vi "抓圓_new.vi"(0 "Image In":T6, 1 "ROI":T5, 4 "Gap":i32=10 min=1 max=300, 5 "error In":errorcluster, 6 "Process":T8(ring), 7 "Options":T3={"Search Direction"=0, "Edge Options"={"Edge Polarity"=0, "Kernel Size"=3, "Width"=3, "Minimum Edge Strength"=10.0, "Interpolation Type"=enum."Bilinear Fixed", "Data Processing Method"=enum."Average"}, "Show Search Area"=FALSE, "Show Search Lines"=FALSE, "Show Edges Found"=FALSE, "Show Result"=TRUE, "Search Area Color"=65280, "Search Lines Color"=255, "Edge Locations Color"=16776960, "Result Color"=16711680, "Overlay Group Name"=""} {"Edge Options"."Edge Polarity" items=["All Edges", "Rising Edges", "Falling Edges"]; "Edge Options"."Minimum Edge Strength" format="%.2f"; "Edge Options"."Width" step=2; "Edge Options"."Kernel Size" step=2; "Search Direction" items=["Outer to Inner", "Inner to Outer"]}, 8 "Point Diameter (5)":u32=5 min=3 max=1000, 10 "Optimized Mode":bool=TRUE) -> (13 "Ellipse":T7 {"Minor Axis"."Point 2"."Y" format="%.2f"; "Minor Axis"."Point 2"."X" format="%.2f"; "Minor Axis"."Point 1"."Y" format="%.2f"; "Minor Axis"."Point 1"."X" format="%.2f"; "Major Axis"."Point 2"."Y" format="%.2f"; "Major Axis"."Point 2"."X" format="%.2f"; "Major Axis"."Point 1"."Y" format="%.2f"; "Major Axis"."Point 1"."X" format="%.2f"; "Center"."Y" format="%.2f"; "Center"."X" format="%.2f"}, 14 "Imag e Out":T6, 15 "Line Profile":dbl[][](graph), 19 "error out":errorcluster)   [LabVIEW 2015]
uses:
  <vilib>/vision/Image Controls.llb/IMAQ Image.ctl
  <vilib>/vision/Measure.llb/Edge Options.ctl
  <vilib>/vision/Measure.llb/Edge Polarity.ctl
  <vilib>/vision/NI_Vision_Development_Module.lvlib
panel:
  in  "Coordinate System":T4 {"Measurement System"."Axis Reference" items=["Direct", "Indirect"]; "Measurement System"."Angle (deg)" format="%.2f"; "Measurement System"."Origin"."Y" format="%.2f"; "Measurement System"."Origin"."X" format="%.2f"; "Reference System"."Axis Reference" items=["Direct", "Indirect"]; "Reference System"."Angle (deg)" format="%.2f"; "Reference System"."Origin"."Y" format="%.2f"; "Reference System"."Origin"."X" format="%.2f"}
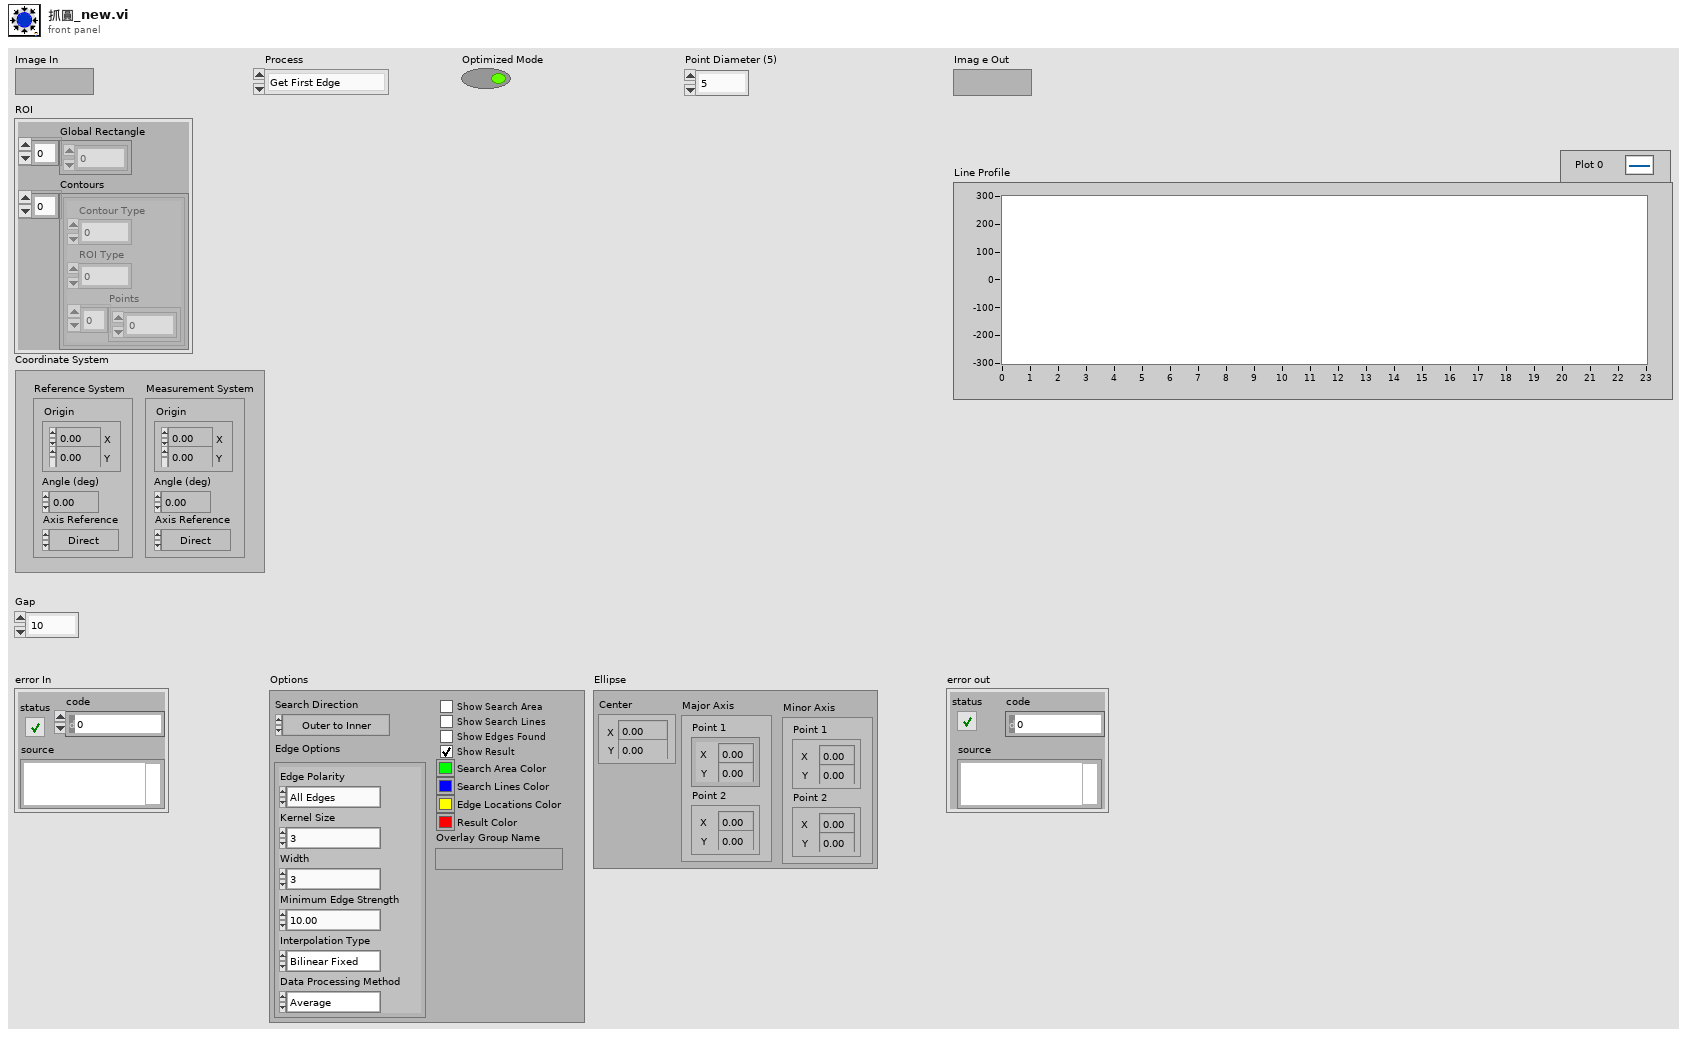
[diagram p1: front panel]
types:
  T1 = typedef "Edge Options.ctl" = cluster{"Edge Polarity":T2, "Kernel Size":u32, "Width":u32, "Minimum Edge Strength":sgl, "Interpolation Type":enum32{"Zero Order", "Bilinear", "Quadratic", "Cubic", "Bilinear Fixed"}, "Data Processing Method":enum32{"Average", "Median"}}
  T2 = typedef "Edge Polarity.ctl" = u32
  T3 = cluster{"Search Direction":u32, "Edge Options":T1, "Show Search Area":bool, "Show Search Lines":bool, "Show Edges Found":bool, "Show Result":bool, "Search Area Color":u32, "Search Lines Color":u32, "Edge Locations Color":u32, "Result Color":u32, "Overlay Group Name":string}
  T4 = typedef "IMAQ Coordinate System" = cluster{"Reference System":cluster{"Origin":cluster{"X":sgl, "Y":sgl}, "Angle (deg)":sgl, "Axis Reference":u32}, "Measurement System":cluster{"Origin":cluster{"X":sgl, "Y":sgl}, "Angle (deg)":sgl, "Axis Reference":u32}}
  T5 = cluster{"Global Rectangle":i32[], "Contours":cluster{"Contour Type":u32, "ROI Type":u32, "Points":i32[]}[]}
  T6 = typedef "IMAQ Image.ctl" = refnum<image>
  T7 = cluster{"Center":cluster{"X":sgl, "Y":sgl}, "Major Axis":cluster{"Point 1":cluster{"X":sgl, "Y":sgl}, "Point 2":cluster{"X":sgl, "Y":sgl}}, "Minor Axis":cluster{"Point 1":cluster{"X":sgl, "Y":sgl}, "Point 2":cluster{"X":sgl, "Y":sgl}}}
  T8 = enum16{"Get First Edge", "Get First + Last Edge", "Get All Edges", "Get Best Edge"}
  T9 = cluster{"Point 1":cluster{"x":dbl, "y":dbl}, "Point 2":cluster{"x":dbl, "y":dbl}}
  T10 = cluster{"Origin":cluster{"X":sgl, "Y":sgl}, "Angle (deg)":sgl, "Axis Reference":u32}
  T11 = typedef "ROI Descriptor" = cluster{"Global Rectangle":i32[], "Contours":cluster{"ID":enum32{"External", "Internal"}, "Type":u32, "Coordinates":i32[]}[]}
  T12 = typedef "Edge New.ctl" = cluster{"Location (Pixel)":cluster{"X":sgl, "Y":sgl}, "Location (Real-World)":cluster{"X":sgl, "Y":sgl}, "Distance (Pixel)":dbl, "Distance (Real-World)":dbl, "Strength":dbl, "Noise":dbl, "Rising?":bool}
  T13 = typedef "Search Line.ctl" = cluster{"Start Point":cluster{"X":sgl, "Y":sgl}, "End Point":cluster{"X":sgl, "Y":sgl}, "Edge Info":T12[], "Edge Map":dbl[], "Calibration Valid":bool}
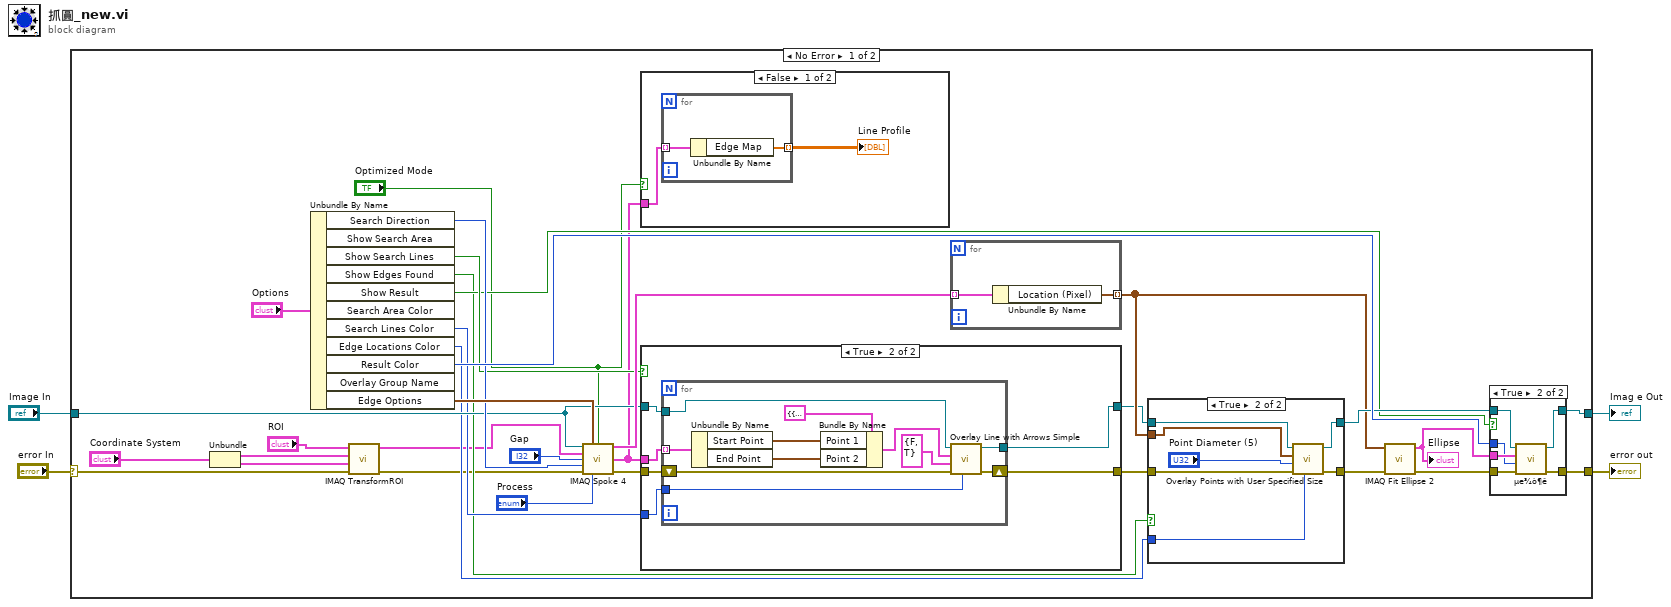
[diagram p0: block diagram]
diagram:
  n1 = case shown="No Error" "error In" {
    selector: "error In" -> [w30 w80]
    tunnel: [w32 w80] -> w4
    tunnel: "Image In" -> [w16 w79]
    tunnel: [w28 w79] -> w1
    frame No Error {
      n2 = Unbundle("Coordinate System") -> ("Reference System"=w35:T10, "Measurement System"=w34:T10)
      n3 = Unbundle By Name("Options") -> ("Search Direction"=w24:u32, "Show Search Lines"=w15:bool, "Show Edges Found"=w11:bool, "Show Result"=w13:bool, "Search Lines Color"=w14:u32, "Edge Locations Color"=w12:u32, "Result Color"=w27:u32, "Edge Options"=w25:T1)  [unwired: 3 out]
      n4 = call "IMAQ TransformROI"("error in (no error)"=w30, "New Reference"=w34, "Base Reference"=w35, "ROI Descriptor"="ROI") -> ("error out"=w10:errorcluster, "ROI Descriptor out"=w9:T11)  [unwired: 6 in]
      n5 = call "IMAQ Spoke 4"("Image"=w16, "Edge Options"=w25, "Optimized Mode"="Optimized Mode", "ROI Descriptor"=w9, "Step Size"="Gap", "Scan Direction"=w24, "error in (no error)"=w10, "Process"="Process") -> ("First Edges"=w26:T12[], "Search Lines"=w5:T13[], "error out"=w22:errorcluster)  [unwired: 4 in, 1 out]
      n6 = case shown="False" "Optimized Mode" {
        tunnel: w5 -> [w38 _]
        frame False {
          n7 = for {
            tunnel: w38 -> [w40] mode=indexing
            tunnel: [w39] -> w37 mode=indexing
            n8 = Unbundle By Name(w40) -> ("Edge Map"=w39:dbl[])
          }
          "Line Profile" <- w37
        }
        frame True {
        }
      }
      n9 = case shown="True" w15 {
        tunnel: w16 -> [w42 w48]
        tunnel: [w42 w47] -> w17
        tunnel: [w41 w46] -> w21
        tunnel: w22 -> [w41 w45]
        tunnel: w14 -> [_ w44]
        tunnel: w5 -> [_ w43]
        frame False {
        }
        frame True {
          n10 = for {
            tunnel: w48 -> [w59]
            tunnel: [w55] -> w47
            tunnel: w44 -> [w52]
            shift-right: [w54] -> w46
            shift-left: w45 -> [w53]
            tunnel: w43 -> [w51] mode=indexing
            n11 = Unbundle By Name(w51) -> ("Start Point"=w50:cluster{"X":sgl, "Y":sgl}, "End Point"=w49:cluster{"X":sgl, "Y":sgl})
            n12 = Bundle By Name(cluster=T9 {"Point 1"={"x"=50.0, "y"=50.0}, "Point 2"={"x"=70.0, "y"=70.0}} ("Line Coordinates"), "Point 1"=w50, "Point 2"=w49) -> (w56:T9)
            n13 = call "Overlay Line with Arrows Simple.vi"("Color"=w52, "error in"=w53, "Arrows"=cluster{"Start point":bool, "End point":bool} {"Start point"=FALSE, "End point"=TRUE}, "Line Coordinates"=w56, "Image In"=w59) -> ("error out"=w54:errorcluster, "Image Out"=w55:T6)  [unwired: 5 in]
          }
        }
      }
      n14 = for {
        tunnel: w26 -> [w70] mode=indexing
        tunnel: [w69] -> w18 mode=indexing
        n15 = Unbundle By Name(w70) -> ("Location (Pixel)"=w69:cluster{"X":sgl, "Y":sgl})
      }
      n16 = case shown="True" w11 {
        tunnel: w21 -> [w60 w68]
        tunnel: w17 -> [w61 w67]
        tunnel: [w61 w66] -> w19
        tunnel: [w60 w65] -> w20
        tunnel: w12 -> [_ w64]
        tunnel: w18 -> [_ w63]
        frame False {
        }
        frame True {
          n17 = call "Overlay Points with User Specified Size.vi"("Color"=w64, "error in"=w68, "Point Diameter (5)"="Point Diameter (5)", "Points"=w63, "Image In"=w67) -> ("error out"=w65:errorcluster, "Image Out"=w66:T6)  [unwired: 5 in]
        }
      }
      n18 = call "IMAQ Fit Ellipse 2"("error in (no error)"=w20, "Radial Points"=w18) -> ("error out"=w31:errorcluster, "Ellipse"=w36:T7)  [unwired: 4 in, 4 out]
      "Ellipse" <- w36
      n19 = case shown="True" w13 {
        tunnel: w36 -> [_ w78]
        tunnel: w19 -> [w72 w77]
        tunnel: [w71 w76] -> w32
        tunnel: w31 -> [w71 w75]
        tunnel: [w72 w74] -> w28
        tunnel: w27 -> [_ w73]
        frame False {
        }
        frame True {
          n20 = call "µe¾ò¶ê.vi"("error in (no error)"=w75, "Color"=w73, "Ellipse"=w78, "Image In"=w77) -> ("error out"=w76:errorcluster, "Image"=w74:T6)  [unwired: 6 in]
        }
      }
    }
    frame Error {
    }
  }
  "error out" <- w4
  "Imag e Out" <- w1
